vi "Log Error Data.vi"(8 "error in":errorcluster, 10 "Error Data":string, 11 "Fault Handler in":refnum<class "Fault Handler.lvclass">) -> (0 "error out":errorcluster, 3 "Fault Handler out":refnum<class "Fault Handler.lvclass">)   [LabVIEW 2019, in "Fault Handler.lvlib" / "Fault Handler.lvclass"]
doc: "This routine is only called when a unique error is generated by the fault handler.\n\nThe error record (generated by the caller) is \n\n 1. Pre-pended with a timestamp of the error occurence\n\n 2. Written to the end of the error report file\n\n 3. Appended to the end of the error log indicator on the fault monitor."
uses:
  Project/Fault Handler.lvclass
  Project/Fault Handler.lvclass/Fault Handler.ctl
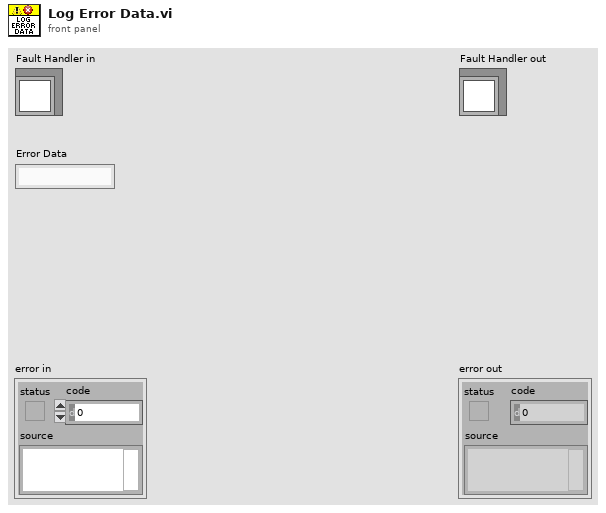
[diagram p1: front panel]
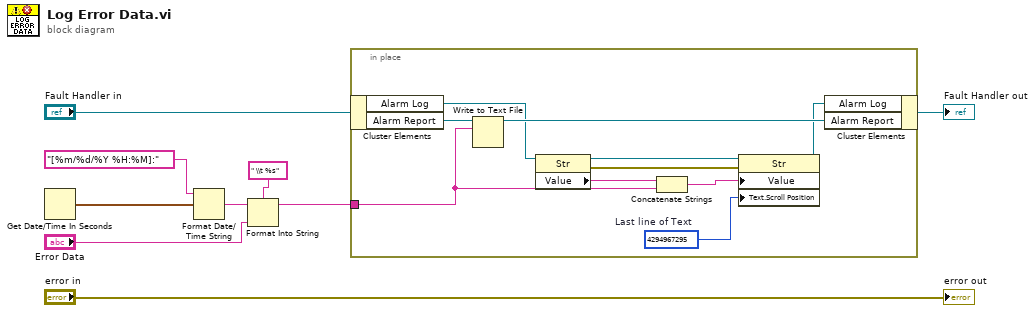
[diagram p0: block diagram]
diagram:
  n1 = Get Date/Time In Seconds() -> (seconds since 1Jan1904=w6:timestamp)
  n2 = Format Date/Time String(time format string (%c)="[%m/%d/%Y %H:%M]:", seconds (now)=w6) -> (date/time string=w8:string)  [unwired: 1 in]
  n3 = Format Into String(format string=" \\t %s", initial string=w8, "Error Data") -> (resulting string=w1:string)  [unwired: 1 in, 1 out]
  n4 = in-place {
    in-place-border: w1 -> [w11]
    w10 = u32 4294967295  # Last line of Text
    n5 = in-place-cluster #1("Fault Handler in") -> ("Alarm Log"=w15:refnum<vi>, "Alarm Report"=w19:refnum<file>)
    n6 = Write to Text File(file (use dialog)=w19, text=w11) -> (refnum out=w18:refnum<file>)  [unwired: 2 in, 2 out]
    n7 = property class="Str"(reference=w15) -> (reference out=w17:refnum<vi>, error out=w16:errorcluster, "Value"=w13:string)  [unwired: 1 in]
    n8 = Concatenate Strings(w13, w11) -> (w12:string)
    n9 = property class="Str"(reference=w17, error in=w16, "Value"=w12, "Text.Scroll Position"=w10) -> (reference out=w14:refnum<vi>)  [unwired: 1 out]
    n10 = in-place-cluster #1("Alarm Log"=w14, "Alarm Report"=w18) -> (→"Fault Handler out":refnum<class "Fault Handler.lvclass">)
  }
  "error out" <- "error in"
